vi "MultiChannel IIR Cascade Filter PtByPt.vi"(7 "initialize":bool, 8 "IIR Filter Cluster":T1, 11 "x":dbl[](array[numeric])) -> (0 "error":i32[](array[numeric]), 3 "Filtered x":dbl[](array[numeric]))   [LabVIEW 2010, in "Filter VIs.lvlib"]
uses:
  <vilib>/Analysis/baseanly.llb/IIR Cascade Filter (DBL).vi
  Filter VIs.lvlib
  <vilib>/Analysis/NI_AALBase.lvlib
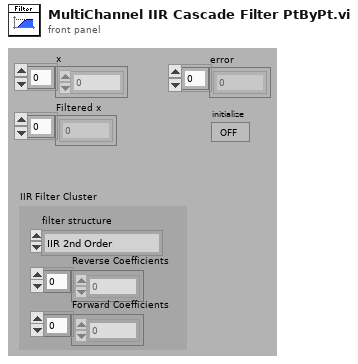
[diagram p1: front panel]
types:
  T1 = cluster{"filter structure":enum32{"IIR 2nd Order", "IIR 4th Order"}, "Reverse Coefficients":dbl[], "Forward Coefficients":dbl[]}
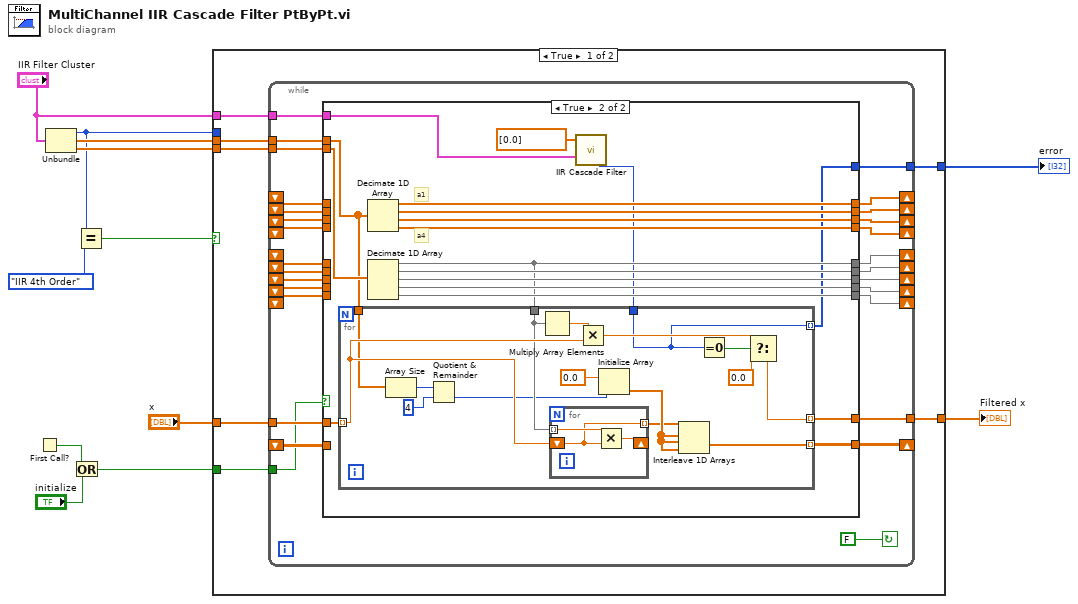
[diagram p0: block diagram]
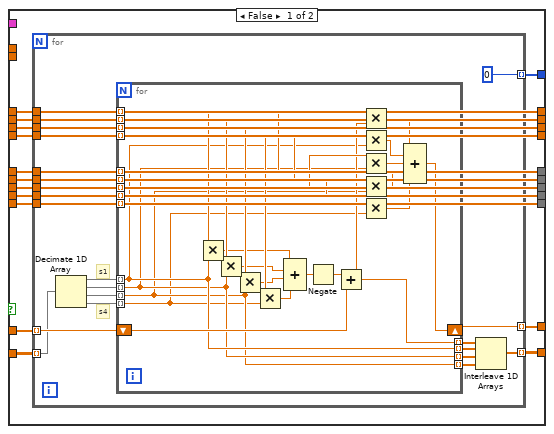
[diagram p2: hidden frame]
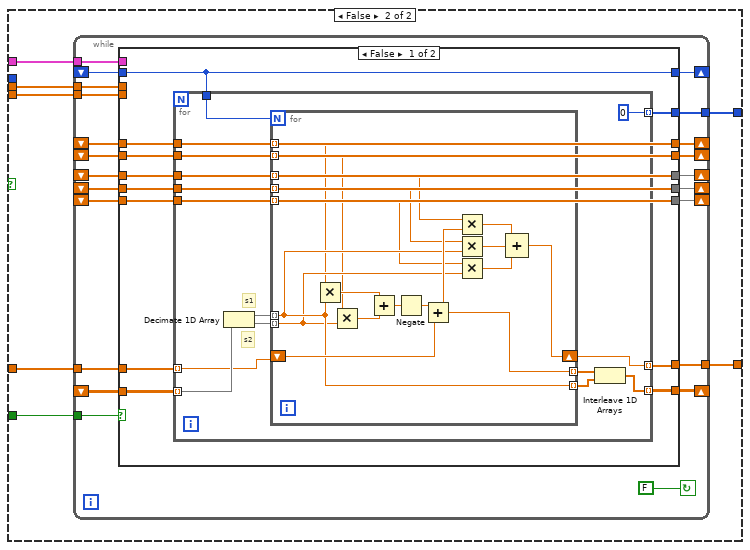
[diagram p3: hidden frame]
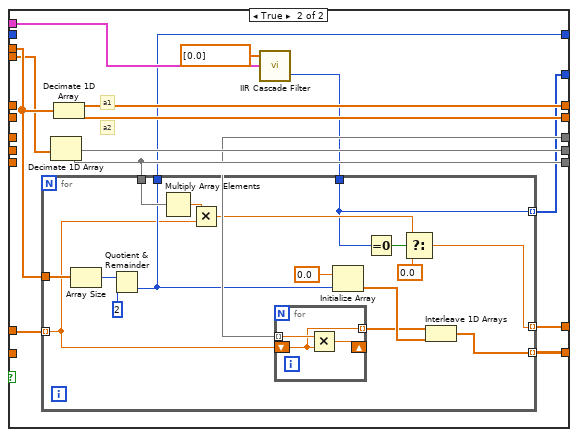
[diagram p4: hidden frame]
diagram:
  n1 = First Call?() -> (First Call?: T/F=w6:bool)
  n2 = Unbundle("IIR Filter Cluster") -> ("filter structure"=w10:enum32{"IIR 2nd Order", "IIR 4th Order"}, "Reverse Coefficients"=w11:dbl[], "Forward Coefficients"=w12:dbl[])
  n3 = Or(x=w6, y="initialize") -> (x .or. y?=w7:bool)
  n4 = Equal?(x=w10, y=enum32{"IIR 2nd Order", "IIR 4th Order"}."IIR 4th Order") -> (x = y?=w8:bool)
  n5 = case shown="True" w8 {
    tunnel: "x" -> [w18 w153]
    tunnel: w12 -> [w16 w151]
    tunnel: w10 -> [_ _]
    tunnel: w11 -> [w17 w152]
    tunnel: [w15 w150] -> w2
    tunnel: w7 -> [w19 w154]
    tunnel: "IIR Filter Cluster" -> [w14 w149]
    tunnel: [w13 w148] -> w1
    frame True {
      n6 = while {
        tunnel: [w21] -> w13
        tunnel: w14 -> [w22]
        tunnel: [w25] -> w15
        shift-left: _ -> [w26]
        shift-right: [w24] -> _
        shift-left: _ -> [w27]
        shift-right: [w28] -> _
        shift-left: _ -> [w29]
        shift-right: [w31] -> _
        shift-left: _ -> [w30]
        shift-right: [w32] -> _
        shift-left: _ -> [w33]
        shift-right: [w34] -> _
        tunnel: w18 -> [w35]
        tunnel: w17 -> [w36]
        shift-left: _ -> [w37]
        shift-right: [w39] -> _
        shift-left: _ -> [w38]
        shift-right: [w40] -> _
        shift-left: _ -> [w42]
        shift-right: [w45] -> _
        shift-left: _ -> [w41]
        shift-right: [w44] -> _
        shift-left: _ -> [w43]
        shift-right: [w46] -> _
        tunnel: w16 -> [w47]
        tunnel: w19 -> [w20]
        stop <- FALSE continue-if-true
        n7 = case shown="True" w20 {
          tunnel: w47 -> [_ w120]
          tunnel: [w56 w124] -> w46
          tunnel: [w55 w123] -> w45
          tunnel: [w54 w122] -> w44
          tunnel: w43 -> [w56 _]
          tunnel: w42 -> [w55 _]
          tunnel: w41 -> [w54 _]
          tunnel: [w59 w126] -> w40
          tunnel: [w58 w125] -> w39
          tunnel: w38 -> [w59 _]
          tunnel: w37 -> [w58 _]
          tunnel: w36 -> [_ w112]
          tunnel: w35 -> [w52 w118]
          tunnel: [w60 w127] -> w34
          tunnel: w33 -> [w60 _]
          tunnel: [w57 w117] -> w32
          tunnel: [w53 w121] -> w31
          tunnel: w30 -> [w57 _]
          tunnel: w29 -> [w53 _]
          tunnel: [w61 w128] -> w28
          tunnel: w27 -> [w61 _]
          tunnel: [w50 w113] -> w25
          tunnel: w26 -> [w51 _]
          tunnel: [w49 w119] -> w24
          tunnel: w22 -> [_ w116]
          tunnel: [w48 w111] -> w21
          frame False {
            n8 = for {
              tunnel: w61 -> [w83]
              tunnel: w60 -> [w82]
              tunnel: w59 -> [w81]
              tunnel: w58 -> [w80]
              tunnel: w57 -> [w79]
              tunnel: w56 -> [w78]
              tunnel: w55 -> [w77]
              tunnel: w54 -> [w76]
              tunnel: w53 -> [w75]
              tunnel: w52 -> [w70] mode=indexing
              tunnel: w51 -> [w69] mode=indexing
              tunnel: [w68] -> w50 mode=indexing
              tunnel: [w63] -> w49 mode=indexing
              tunnel: [0 ("error")] -> w48 mode=indexing
              # "s4"
              # "s1"
              n9 = Decimate 1D Array(w69) -> (w74:dbl[], w73:dbl[], w72:dbl[], w71:dbl[])
              n10 = for {
                tunnel: w81 -> [w108] mode=indexing
                tunnel: w80 -> [w107] mode=indexing
                tunnel: w78 -> [w99] mode=indexing
                tunnel: w77 -> [w98] mode=indexing
                tunnel: w76 -> [w97] mode=indexing
                tunnel: w82 -> [w109] mode=indexing
                tunnel: w75 -> [w96] mode=indexing
                tunnel: w83 -> [w110] mode=indexing
                tunnel: w79 -> [w100] mode=indexing
                tunnel: w74 -> [w87] mode=indexing
                tunnel: w73 -> [w86] mode=indexing
                tunnel: w72 -> [w85] mode=indexing
                tunnel: w71 -> [w84] mode=indexing
                tunnel: [w88] -> w67 mode=indexing
                tunnel: [w85] -> w64 mode=indexing
                tunnel: [w86] -> w65 mode=indexing
                tunnel: [w87] -> w66 mode=indexing
                shift-right: [w89] -> w68
                shift-left: w70 -> [w90]
                n11 = Multiply(x=w110, y=w87) -> (x*y=w106:dbl)
                n12 = Multiply(x=w109, y=w86) -> (x*y=w105:dbl)
                n13 = Multiply(x=w108, y=w85) -> (x*y=w104:dbl)
                n14 = Multiply(x=w107, y=w84) -> (x*y=w103:dbl)
                n15 = Compound Arithmetic op=ADD(w106, w105, w104, w103) -> (w102:dbl)
                n16 = Negate(x=w102) -> (-x=w101:dbl)
                n17 = Add(x=w101, y=w90) -> (x+y=w88:dbl)
                n18 = Multiply(x=w100, y=w88) -> (x*y=w95:dbl)
                n19 = Multiply(x=w99, y=w87) -> (x*y=w94:dbl)
                n20 = Multiply(x=w98, y=w86) -> (x*y=w93:dbl)
                n21 = Multiply(x=w97, y=w85) -> (x*y=w92:dbl)
                n22 = Multiply(x=w96, y=w84) -> (x*y=w91:dbl)
                n23 = Compound Arithmetic op=ADD(w95, w94, w93, w92, w91) -> (w89:dbl)
              }
              n24 = Interleave 1D Arrays(w67, w66, w65, w64) -> (w63:dbl[])
            }
          }
          frame True {
            # "a4"
            # "a1"
            n25 = Decimate 1D Array(w112) -> (w128:dbl[], w127:dbl[], w126:dbl[], w125:dbl[])
            n26 = Decimate 1D Array(w120) -> (w117:dbl[], w124:dbl[], w123:dbl[], w122:dbl[], w121:dbl[])
            n27 = call-poly <vilib>:"IIR Cascade Filter.vi"("IIR Filter Cluster"=w116, "X"=dbl[] [0.0]) -> ("error"=w114:i32)  [unwired: 1 in, 1 out]
            n28 = for {
              tunnel: [w141] -> w119 mode=indexing
              tunnel: w118 -> [w140] mode=indexing
              tunnel: w117 -> [w139]
              tunnel: w114 -> [w129]
              tunnel: [w135] -> w113 mode=indexing
              tunnel: w112 -> [w133]
              tunnel: [w129] -> w111 mode=indexing
              n29 = Array Size(array=w133) -> (size(s)=w132:i32)
              n30 = Quotient & Remainder(x=w132, y=4) -> (floor(x/y)=w130:i32)  [unwired: 1 out]
              n31 = Multiply Array Elements(1:w139) -> (0:w144:dbl)
              n32 = for {
                shift-right: [w146] -> _
                shift-left: w140 -> [w145]
                tunnel: w139 -> [w147] mode=indexing
                tunnel: [w145] -> w138 mode=indexing
                n33 = Multiply(x=w147, y=w145) -> (x*y=w146:dbl)
              }
              n34 = Multiply(x=w144, y=w140) -> (x*y=w136:dbl)
              n35 = Initialize Array(0.0 ("Element Data"), w130) -> (w142:dbl[])
              n36 = Interleave 1D Arrays(w138, w142, w142, w142) -> (w141:dbl[])
              n37 = Equal To 0?(x=w129) -> (x = 0?=w137:bool)
              n38 = Select(t=w136, s=w137, f=0.0) -> (s? t:f=w135:dbl)
            }
          }
        }
      }
    }
    frame False {
      n39 = while {
        tunnel: [w156] -> w148
        tunnel: w149 -> [w157]
        tunnel: [w160] -> w150
        shift-left: _ -> [w161]
        shift-right: [w159] -> _
        shift-left: _ -> [w164]
        shift-right: [w165] -> _
        shift-left: _ -> [w166]
        shift-right: [w167] -> _
        shift-left: _ -> [w168]
        shift-right: [w169] -> _
        tunnel: w153 -> [w170]
        tunnel: w152 -> [w171]
        shift-left: _ -> [w172]
        shift-right: [w174] -> _
        shift-left: _ -> [w173]
        shift-right: [w175] -> _
        shift-left: _ -> [w162]
        shift-right: [w163] -> _
        tunnel: w151 -> [w176]
        tunnel: w154 -> [w155]
        stop <- FALSE continue-if-true
        n40 = case shown="False" w155 {
          tunnel: w176 -> [_ w224]
          tunnel: [w184 w232] -> w175
          tunnel: [w183 w231] -> w174
          tunnel: w173 -> [w184 _]
          tunnel: w172 -> [w183 _]
          tunnel: w171 -> [_ w229]
          tunnel: w170 -> [w178 w223]
          tunnel: [w181 w233] -> w169
          tunnel: w168 -> [w181 _]
          tunnel: [w185 w228] -> w167
          tunnel: w166 -> [w185 _]
          tunnel: [w182 w234] -> w165
          tunnel: w164 -> [w182 _]
          tunnel: [w186 w225] -> w163
          tunnel: w162 -> [w186 _]
          tunnel: [w179 w221] -> w160
          tunnel: w161 -> [w187 _]
          tunnel: [w180 w230] -> w159
          tunnel: w157 -> [_ w227]
          tunnel: [w177 w220] -> w156
          frame False {
            n41 = for {
              tunnel: w187 -> [w202] mode=indexing
              tunnel: w186 -> [w201]
              tunnel: w185 -> [w200]
              tunnel: w184 -> [w199]
              tunnel: w183 -> [w198]
              tunnel: w182 -> [w197]
              tunnel: w181 -> [w196]
              tunnel: [w191] -> w180 mode=indexing
              tunnel: [w190] -> w179 mode=indexing
              tunnel: w178 -> [w189] mode=indexing
              tunnel: [0 ("error")] -> w177 mode=indexing
              # "s2"
              # "s1"
              n42 = Decimate 1D Array(w202) -> (w195:dbl[], w194:dbl[])
              n43 = for {
                N: w201 -> [_]
                tunnel: w195 -> [w209] mode=indexing
                tunnel: w194 -> [w208] mode=indexing
                tunnel: [w210] -> w193 mode=indexing
                tunnel: [w209] -> w192 mode=indexing
                shift-right: [w211] -> w190
                shift-left: w189 -> [w212]
                tunnel: w200 -> [w207] mode=indexing
                tunnel: w199 -> [w206] mode=indexing
                tunnel: w198 -> [w205] mode=indexing
                tunnel: w197 -> [w204] mode=indexing
                tunnel: w196 -> [w203] mode=indexing
                n44 = Multiply(x=w204, y=w209) -> (x*y=w219:dbl)
                n45 = Multiply(x=w203, y=w208) -> (x*y=w218:dbl)
                n46 = Add(x=w219, y=w218) -> (x+y=w217:dbl)
                n47 = Negate(x=w217) -> (-x=w216:dbl)
                n48 = Add(x=w216, y=w212) -> (x+y=w210:dbl)
                n49 = Multiply(x=w207, y=w210) -> (x*y=w215:dbl)
                n50 = Multiply(x=w206, y=w209) -> (x*y=w214:dbl)
                n51 = Multiply(x=w205, y=w208) -> (x*y=w213:dbl)
                n52 = Compound Arithmetic op=ADD(w215, w214, w213) -> (w211:dbl)
              }
              n53 = Interleave 1D Arrays(w193, w192) -> (w191:dbl[])
            }
          }
          frame True {
            # "a2"
            # "a1"
            n54 = Decimate 1D Array(w224) -> (w228:dbl[], w232:dbl[], w231:dbl[])
            n55 = Decimate 1D Array(w229) -> (w234:dbl[], w233:dbl[])
            n56 = call-poly <vilib>:"IIR Cascade Filter.vi"("IIR Filter Cluster"=w227, "X"=dbl[] [0.0]) -> ("error"=w222:i32)  [unwired: 1 in, 1 out]
            n57 = for {
              tunnel: [w247] -> w230 mode=indexing
              tunnel: w229 -> [w246]
              tunnel: w228 -> [w244]
              tunnel: [w242] -> w225
              tunnel: w223 -> [w240] mode=indexing
              tunnel: w222 -> [w235]
              tunnel: [w236] -> w221 mode=indexing
              tunnel: [w235] -> w220 mode=indexing
              n58 = Array Size(array=w246) -> (size(s)=w241:i32)
              n59 = Quotient & Remainder(x=w241, y=2) -> (floor(x/y)=w242:i32)  [unwired: 1 out]
              n60 = Multiply Array Elements(1:w244) -> (0:w250:dbl)
              n61 = Multiply(x=w250, y=w240) -> (x*y=w238:dbl)
              n62 = for {
                shift-right: [w252] -> _
                shift-left: w240 -> [w251]
                tunnel: w244 -> [w253] mode=indexing
                tunnel: [w251] -> w243 mode=indexing
                n63 = Multiply(x=w253, y=w251) -> (x*y=w252:dbl)
              }
              n64 = Initialize Array(0.0 ("Element Data"), w242) -> (w245:dbl[])
              n65 = Equal To 0?(x=w235) -> (x = 0?=w239:bool)
              n66 = Select(t=w238, s=w239, f=0.0) -> (s? t:f=w236:dbl)
              n67 = Interleave 1D Arrays(w243, w245) -> (w247:dbl[])
            }
          }
        }
      }
    }
  }
  "error" <- w1
  "Filtered x" <- w2
